vi "Bitfile.Download.vi"(8 "error in (no error)":errorcluster, 10 "Resource":string, 11 "path":path) -> (0 "error out":errorcluster, 5 "FPGA Session":u32)   [LabVIEW 2019, in "Diagnostics Addon Engine.lvlib"]
uses:
  Diagnostics Addon Engine.lvlib
  <vilib>/rvi/Utilities/XML/nirviXML_GetValue_String.vi
  NiFpga.dll
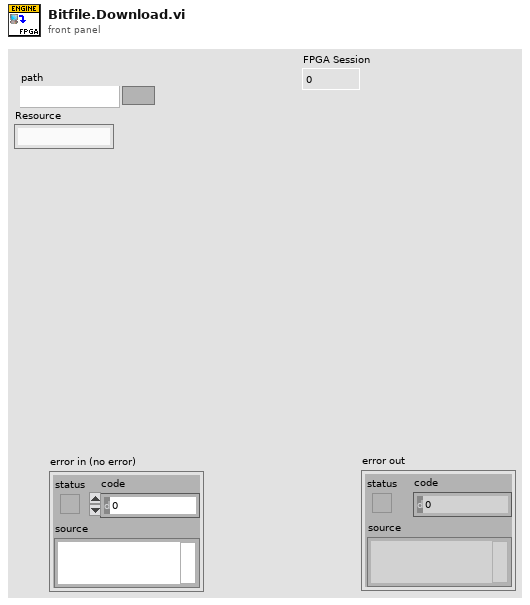
[diagram p1: front panel]
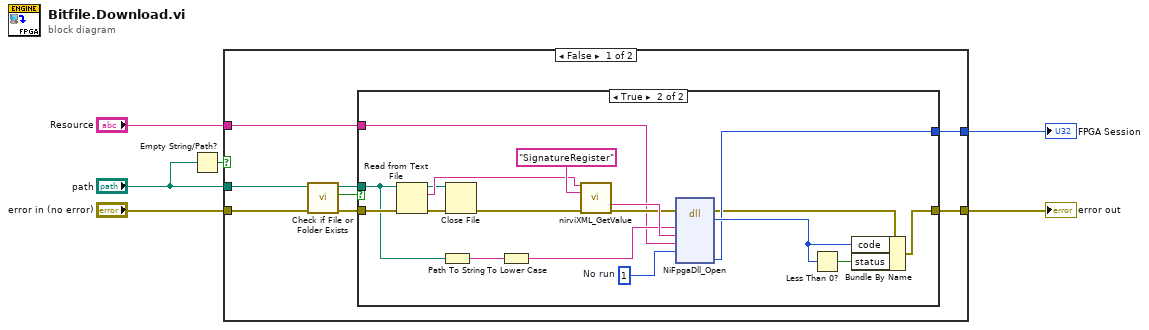
[diagram p0: block diagram]
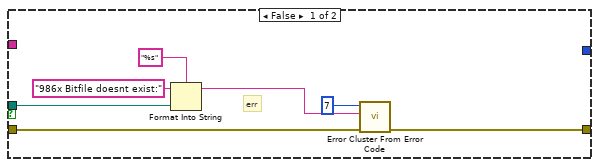
[diagram p2: hidden frame]
diagram:
  n1 = Empty String/Path?(string/path="path") -> (empty?=w3:bool)
  n2 = case shown="False" w3 {
    tunnel: "error in (no error)" -> [w13 w40]
    tunnel: [w14 w40] -> w5
    tunnel: "path" -> [w7 _]
    tunnel: "Resource" -> [w9 _]
    tunnel: [w8 _] -> w4
    frame False {
      n3 = call <vilib>:"Check if File or Folder Exists.vi"("error in (no error)"=w13, "path"=w7) -> ("error out"=w12:errorcluster, "file or folder exists?"=w11:bool, "dup path"=w10:path)  [unwired: 7 in]
      n4 = case shown="True" w11 {
        tunnel: [w16 w36] -> w14
        tunnel: w12 -> [w18 w29]
        tunnel: w10 -> [w21 w28]
        tunnel: w9 -> [_ w22]
        tunnel: [_ w26] -> w8
        frame False {
          # "err"
          n5 = Format Into String(format string="%s", initial string="986x Bitfile doesnt exist:", w21) -> (resulting string=w17:string)  [unwired: 1 in, 1 out]
          n6 = call <vilib>:"Error Cluster From Error Code.vi"("error in (no error)"=w18, "error message (\"\")"=w17, "error code (0)"=7) -> ("error out"=w16:errorcluster)  [unwired: 1 in, 5 out]
        }
        frame True {
          w35 = u32 1  # No run
          n7 = Read from Text File(file (use dialog)=w28, error in=w29) -> (refnum out=w32:refnum<file>, text=w33:string, error out=w31:errorcluster)  [unwired: 3 out]
          n8 = Path To String(path=w28) -> (string=w39:string)
          n9 = Close File(refnum=w32, error in=w31) -> (error out=w30:errorcluster)  [unwired: 1 out]
          n10 = To Lower Case(string=w39) -> (all lower case string=w23:string)
          n11 = call-poly <vilib>:"nirviXML_GetValue.vi"("xml string in"=w33, "tag name in"="SignatureRegister" ("tag"), "error in (no error)"=w30) -> ("value"=w27:string, "error out"=w25:errorcluster)  [unwired: 2 in, 9 out]
          n12 = dll-call lib="NiFpga.*" fn="NiFpgaDll_Open"(error in=w25, "Bitfile"=w23, "Signature"=w27, "Resource"=w22, "Attribute"=w35) -> (error out=w24:errorcluster, "Status"=w37:i32, "Session"=w26:u32)  [unwired: 7 in, 1 out]
          n13 = Less Than 0?(x=w37) -> (x < 0?=w38:bool)
          n14 = Bundle By Name(cluster=w24, "code"=w37, "status"=w38) -> (w36:errorcluster)
        }
      }
    }
    frame True {
    }
  }
  "error out" <- w5
  "FPGA Session" <- w4
